vi "controlNSteps.vi"(5 "set":bool=TRUE, 7 "FWD":bool=TRUE, 8 "error in":errorcluster, 9 "setnSteps in":i32=1, 10 "axis in":u8, 11 "connection ID":i32) -> (0 "error out":errorcluster, 1 "setnSteps out":i32, 2 "axis out":u8, 3 "connection ID":i32)   [LabVIEW 2016]
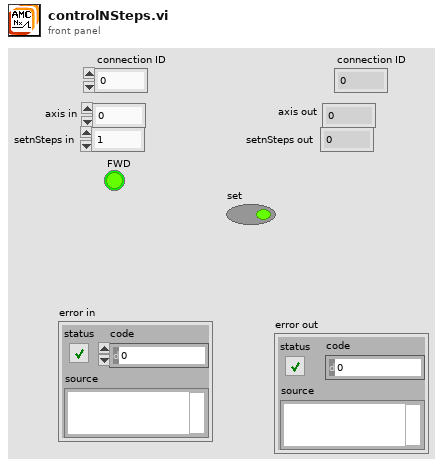
[diagram p1: front panel]
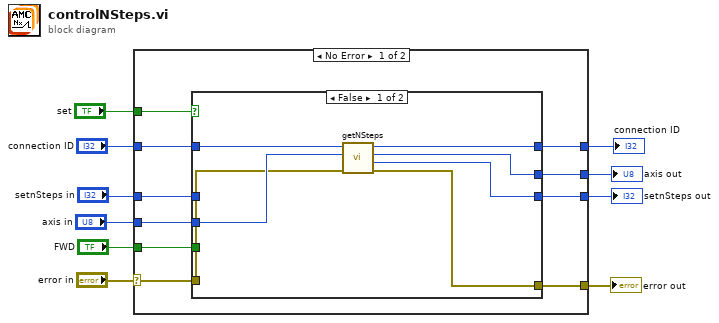
[diagram p0: block diagram]
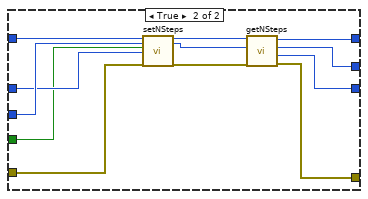
[diagram p2: hidden frame]
diagram:
  n1 = case shown="No Error" "error in" {
    selector: "error in" -> [w12 w40]
    tunnel: "axis in" -> [w17 w43]
    tunnel: [w11 w40] -> w9
    tunnel: [w14 w43] -> w8
    tunnel: "setnSteps in" -> [w15 w42]
    tunnel: [w18 w41] -> w6
    tunnel: "connection ID" -> [w19 w41]
    tunnel: "FWD" -> [w16 _]
    tunnel: [w13 w42] -> w2
    tunnel: "set" -> [w20 _]
    frame No Error {
      n2 = case shown="False" w20 {
        tunnel: w19 -> [w27 w39]
        tunnel: [w26 w33] -> w18
        tunnel: w17 -> [w25 w38]
        tunnel: w16 -> [_ w35]
        tunnel: w15 -> [_ w37]
        tunnel: [w24 w30] -> w14
        tunnel: [w23 w29] -> w13
        tunnel: w12 -> [w22 w36]
        tunnel: [w21 w28] -> w11
        frame False {
          n3 = call "getNSteps.vi"("error in"=w22, "axis"=w25, "connection ID"=w27) -> ("error out"=w21:errorcluster, "nbrstep"=w23:i32, "axis_out"=w24:i32, "connection ID"=w26:i32)  [unwired: 5 in]
        }
        frame True {
          n4 = call "setNSteps.vi"("connection ID"=w39, "axis"=w38, "backward"=w35, "step"=w37, "error in"=w36) -> ("connection ID"=w34:i32, "axis_out"=w32:i32, "error out"=w31:errorcluster)  [unwired: 12 in]
          n5 = call "getNSteps.vi"("error in"=w31, "axis"=w32, "connection ID"=w34) -> ("error out"=w28:errorcluster, "nbrstep"=w29:i32, "axis_out"=w30:i32, "connection ID"=w33:i32)  [unwired: 5 in]
        }
      }
    }
    frame Error {
    }
  }
  "error out" <- w9
  "axis out" <- w8
  "setnSteps out" <- w2
  "connection ID" <- w6
